vi "comicvine.to.local_storyArc.vi"(8 "error in (no error)":errorcluster, 11 "cv storyArc":T1) -> (0 "error out":errorcluster, 3 "local storyArc":T5)   [LabVIEW 2024]
uses:
  <userlib>/_OpenG.lib/string/string.llb/openg_string.lvlib
  definitions/local_storyArc.ctl
  definitions/comicvine_volume.publisher.ctl
  definitions/comicvine_volume.issue.ctl
  definitions/comicvine_volume.results.ctl
  definitions/comicvine_storyArc.ctl
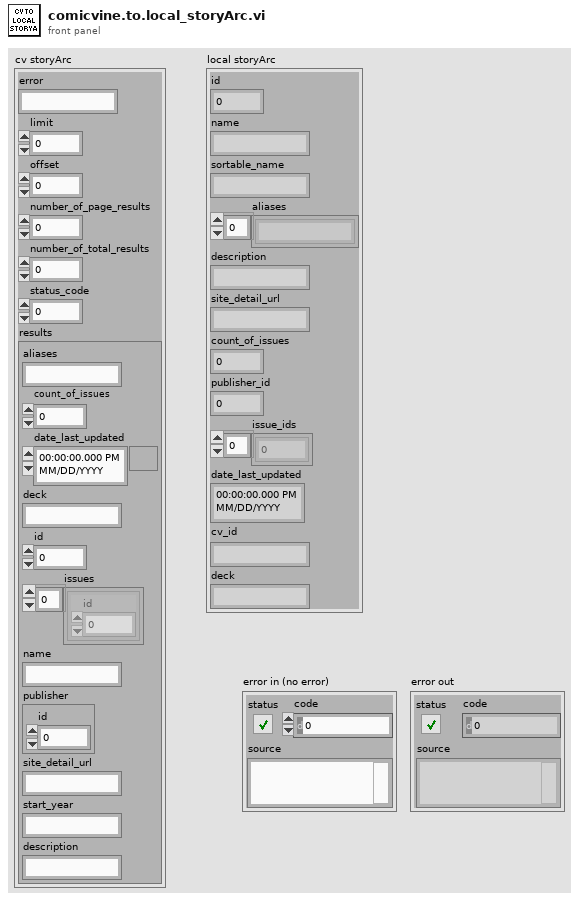
[diagram p1: front panel]
types:
  T1 = typedef "comicvine_storyArc.ctl" = cluster{"error":string, "limit":i32, "offset":i32, "number_of_page_results":i32, "number_of_total_results":i32, "status_code":i32, "results":T2}
  T2 = typedef "comicvine_volume.results.ctl" = cluster{"aliases":string, "count_of_issues":i32, "date_last_updated":timestamp, "deck":string, "id":i32, "issues":T3[], "name":string, "publisher":T4, "site_detail_url":string, "start_year":string, "description":string}
  T3 = typedef "comicvine_volume.issue.ctl" = cluster{"id":i32}
  T4 = typedef "comicvine_volume.publisher.ctl" = cluster{"id":i32}
  T5 = typedef "local_storyArc.ctl" = cluster{"id":i32, "name":string, "sortable_name":string, "aliases":string[], "description":string, "site_detail_url":string, "count_of_issues":i32, "publisher_id":i32, "issue_ids":i32[], "date_last_updated":timestamp, "cv_id":string, "deck":string}
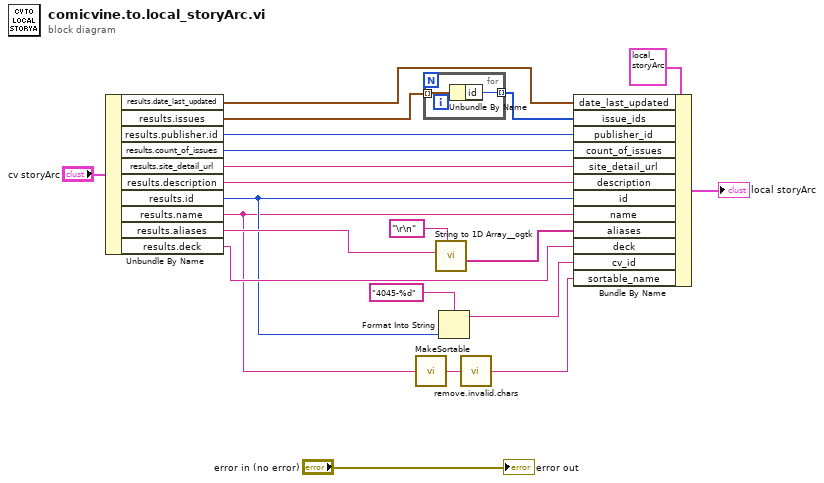
[diagram p0: block diagram]
diagram:
  n1 = Unbundle By Name("cv storyArc") -> ("results.date_last_updated"=w8:timestamp, "results.issues"=w10:T3[], "results.publisher.id"=w11:i32, "results.count_of_issues"=w12:i32, "results.site_detail_url"=w13:string, "results.description"=w14:string, "results.id"=w5:i32, "results.name"=w2:string, "results.aliases"=w17:string, "results.deck"=w7:string)
  n2 = call "MakeSortable.vi"("string in"=w2) -> ("string out"=w18:string)
  n3 = for {
    tunnel: w10 -> [w23] mode=indexing
    tunnel: [w22] -> w9 mode=indexing
    n4 = Unbundle By Name(w23) -> ("id"=w22:i32)
  }
  n5 = call <userlib>:"String to 1D Array__ogtk.vi"("delimiter (Tab)"="\r\n", "string"=w17) -> ("Array of Strings"=w15:string[])  [unwired: 9 in]
  n6 = Format Into String(format string="4045-%d", w5) -> (resulting string=w4:string)  [unwired: 2 in, 1 out]
  n7 = call "remove.invalid.chars.vi"("string in"=w18) -> ("string out"=w1:string)
  n8 = Bundle By Name(cluster=T5 {"id"=0, "name"="", "sortable_name"="", "aliases"=[], "description"="", "site_detail_url"="", "count_of_issues"=0, "publisher_id"=0, "issue_ids"=[], "date_last_updated"=timestamp(0 s since 1904-01-01), "cv_id"="", "deck"=""} ("storyArc"), "date_last_updated"=w8, "issue_ids"=w9, "publisher_id"=w11, "count_of_issues"=w12, "site_detail_url"=w13, "description"=w14, "id"=w5, "name"=w2, "aliases"=w15, "deck"=w7, "cv_id"=w4, "sortable_name"=w1) -> (→"local storyArc":T5)
  "error out" <- "error in (no error)"
